vi "Swerve Rotation Math.vi"(9 "Wheel Speed":dbl, 10 "Wheel Angle":dbl, 11 "Encoder":dbl) -> (0 "Goal":dbl, 2 "Wheel Speed":dbl, 3 "Difference":dbl)   [LabVIEW 2020]
panel:
  # "Goal Angle"
  # "Input"
  # "Difference in degrees"
  # "Current Angle"
  # "Difference in Radians"
  # "Output"
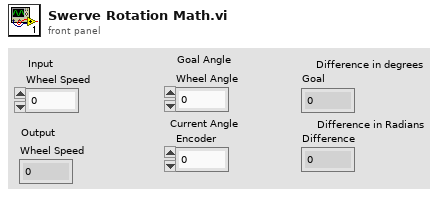
[diagram p1: front panel]
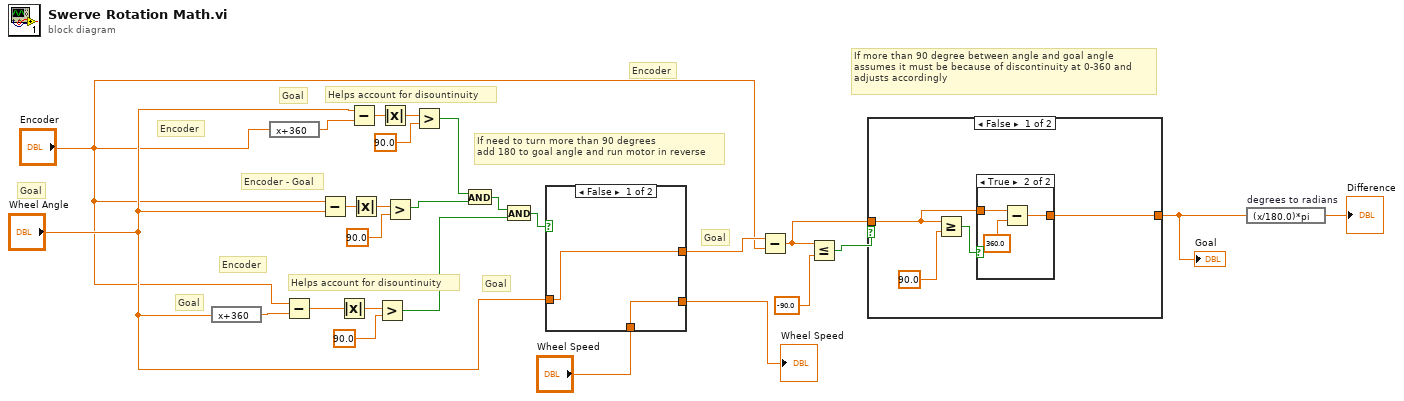
[diagram p0: block diagram]
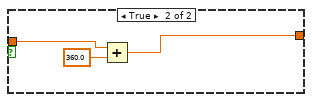
[diagram p3: hidden frame]
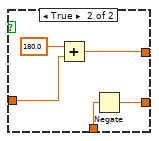
[diagram p4: hidden frame]
diagram:
  # "Helps account for disountinuity"
  # "Helps account for disountinuity"
  # "Encoder"
  # "Goal"
  # "Goal"
  # "Goal"
  # "Encoder"
  # "Goal"
  # "Goal"
  # "Encoder"
  # "Encoder - Goal"
  # "If more than 90 degree between angle and goal angle\nassumes it must be because of discontinuity at 0-360 and\nadjusts accordingly"
  # "If need to turn more than 90 degrees\nadd 180 to goal angle and run motor in reverse"
  n1 = expression code="x+360"("Wheel Angle") -> (w6:dbl)
  n2 = expression code="x+360"("Encoder") -> (w7:dbl)
  n3 = Subtract(x="Encoder", y=w6) -> (x-y=w25:dbl)
  n4 = Subtract(x="Encoder", y="Wheel Angle") -> (x-y=w20:dbl)
  n5 = Absolute Value(x=w25) -> (abs(x)=w24:dbl)
  n6 = Subtract(x="Wheel Angle", y=w7) -> (x-y=w26:dbl)
  n7 = Absolute Value(x=w20) -> (abs(x)=w19:dbl)
  n8 = Greater?(x=w24, y=90.0) -> (0:w16:bool)
  n9 = Absolute Value(x=w26) -> (abs(x)=w22:dbl)
  n10 = Greater?(x=w19, y=90.0) -> (0:w14:bool)
  n11 = Greater?(x=w22, y=90.0) -> (0:w13:bool)
  n12 = And(x=w13, y=w14) -> (x .and. y?=w15:bool)
  n13 = And(x=w15, y=w16) -> (x .and. y?=w17:bool)
  n14 = case shown="False" w17 {
    tunnel: "Wheel Angle" -> [w28 w33]
    tunnel: [w28 w31] -> w12
    tunnel: "Wheel Speed" -> [w27 w30]
    tunnel: [w27 w29] -> w1
    frame False {
    }
    frame True {
      n15 = Add(x=180.0, y=w33) -> (x+y=w31:dbl)
      n16 = Negate(x=w30) -> (-x=w29:dbl)
    }
  }
  "Wheel Speed" <- w1
  n17 = Subtract(x=w12, y="Encoder") -> (x-y=w9:dbl)
  n18 = Less Or Equal?(x=w9, y=-90.0) -> (x <= y?=w10:bool)
  n19 = case shown="False" w10 {
    tunnel: [w34 w43] -> w8
    tunnel: w9 -> [w35 w42]
    frame False {
      n20 = Greater Or Equal?(x=w35, y=90.0) -> (x >= y?=w36:bool)
      n21 = case shown="True" w36 {
        tunnel: w35 -> [w38 w41]
        tunnel: [w38 w40] -> w34
        frame False {
        }
        frame True {
          n22 = Subtract(x=w41, y=360.0) -> (x-y=w40:dbl)
        }
      }
    }
    frame True {
      n23 = Add(x=w42, y=360.0) -> (x+y=w43:dbl)
    }
  }
  "Goal" <- w8
  n24 = expression code="(x/180.0)*pi" "degrees to radians"(w8) -> (→"Difference":dbl)
